vi "TCP_Cliente.vi"() -> ()   [LabVIEW 2020]
uses:
  <vilib>/ErrorRing/Error Ring.xnode
panel:
  in  "Puerto":u16
  in  "stop":bool
  in  "String":string
  out "Tamaño data TCP":i32
  out "length":i32
  out "*(type *) &x":string
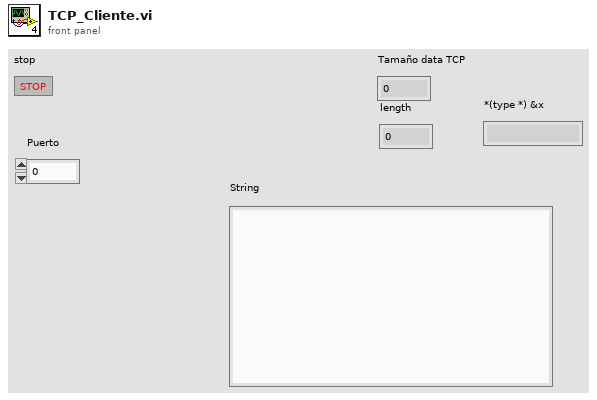
[diagram p1: front panel]
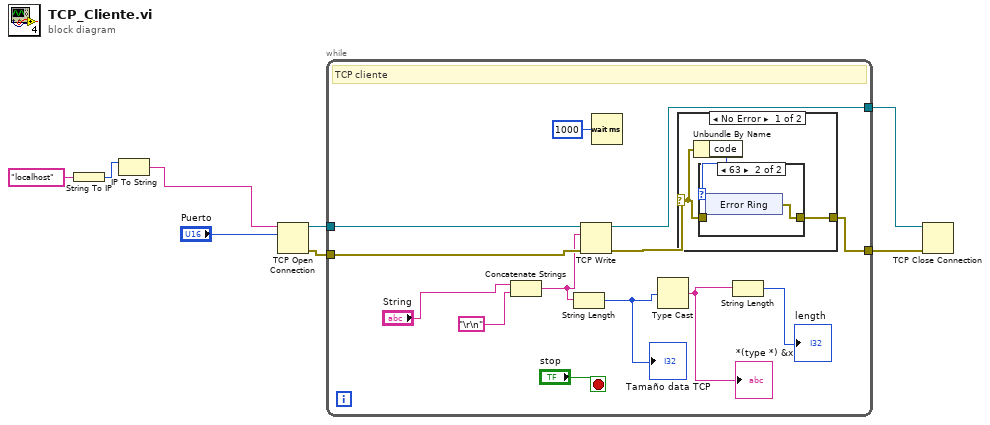
[diagram p0: block diagram]
diagram:
  n1 = String To IP(1:"localhost" ("name")) -> (0:w3:u32)
  n2 = IP To String(2:w3) -> (0:w4:string)  [unwired: 1 in]
  n3 = TCP Open Connection(address=w4, remote port or service name="Puerto") -> (connection ID=w8:refnum<k5>, error out=w7:errorcluster)  [unwired: 3 in]
  n4 = while {
    tunnel: w8 -> [w20]
    tunnel: w7 -> [w19]
    tunnel: [w11] -> w5
    tunnel: [w10] -> w1
    stop <- "stop" stop-if-true
    # "TCP cliente"
    n5 = Concatenate Strings("String", "\r\n") -> (w16:string)
    n6 = String Length(string=w16) -> (length=w15:i32)
    "Tamaño data TCP" <- w15
    n7 = TCP Write(connection ID=w20, data in=w16, error in (no error)=w19) -> (connection ID out=w10:refnum<k5>, error out=w12:errorcluster)  [unwired: 1 in, 1 out]
    n8 = Wait (ms)(milliseconds to wait=u32 1000) -> ()  [unwired: 1 out]
    n9 = Type Cast(x=w15) -> (*(type *) &x=w14:string)  [unwired: 1 in]
    "*(type *) &x" <- w14
    n10 = case shown="No Error" w12 {
      selector: w12 -> [w23 w28]
      tunnel: [w24 w28] -> w11
      frame No Error {
        n11 = Unbundle By Name(w23) -> ("code"=w22:i32)
        n12 = case shown="63" w22 {
          tunnel: [w25 w26] -> w24
          tunnel: w23 -> [w25 _]
          frame 0, Default {
          }
          frame 63 {
            n13 = xnode "Error Ring"() -> ("error out"=w26:errorcluster)
          }
        }
      }
      frame Error {
      }
    }
    n14 = String Length(string=w14) -> (length=→"length":i32)
  }
  n15 = TCP Close Connection(connection ID=w1, error in (no error)=w5) -> ()  [unwired: 1 in, 2 out]
